vi "Obtain Broadcast Events.vi"(8 "error in (no error)":errorcluster, 10 "Create New? (F)":bool) -> (0 "error out":errorcluster, 2 "CE14_v2 Broadcast Events":T1)   [LabVIEW 2018, in "CE14_v2.lvlib"]
doc: "This VI Obtains/Creates the Broadcast events that will be used for other modules to register to receive messages from the module that owns this VI.\n\n<b>NOTE</b>: The contents of this VI are automatically generated and modified by the <b>Tools > Delacor > DQMH</b> utilities. Consider using those utilities instead of making your own modifications to this VI.\n_____\nBased on DQMH Project Template 6.0.0.91."
uses:
  CE14_v2.lvlib
  Broadcast Events--cluster.ctl
  Did Init Argument--cluster.ctl
  Status Updated Argument--cluster.ctl
  Error Reported Argument--cluster.ctl
  Stop Argument--cluster.ctl
  Get Module Execution Status Argument--cluster.ctl
  CE14 response data Argument--cluster.ctl
  Instrument Drivers/LVdriver_CE14(eMIC)/type defs/CE14.data.ctl
  Instrument Drivers/LVdriver_CE14(eMIC)/CE14_eMIC.lvlib
panel:
  # "NOTE: The contents of this VI are automatically generated and modified by the Tools > Delacor > DQMH utilities. Consider using those utilities instead of making your own modifications to this VI."
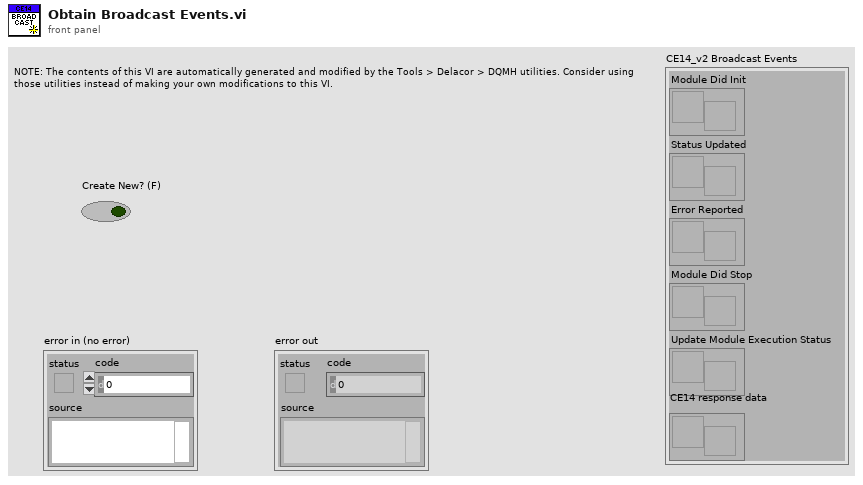
[diagram p1: front panel]
types:
  T1 = typedef "CE14_v2.lvlib/Broadcast Events--cluster.ctl" = cluster{"Module Did Init":refnum<user-event>, "Status Updated":refnum<user-event>, "Error Reported":refnum<user-event>, "Module Did Stop":refnum<user-event>, "Update Module Execution Status":refnum<user-event>, "CE14 response data":refnum<user-event>}
  T2 = typedef "CE14_v2.lvlib/CE14 response data Argument--cluster.ctl" = cluster{"Module ID":i32, "Array":T3[]}
  T3 = typedef "CE14_eMIC.lvlib/CE14.data.ctl" = cluster{"string":string, "float":dbl, "Name":string}
  T4 = typedef "CE14_v2.lvlib/Get Module Execution Status Argument--cluster.ctl" = cluster{"Module ID":i32, "Running?":bool}
  T5 = typedef "CE14_v2.lvlib/Stop Argument--cluster.ctl" = cluster{"Module ID":i32, "Origin":string, "Exit via Stop Module Req?":bool, "Wait for Module to stop?":bool}
  T6 = typedef "CE14_v2.lvlib/Error Reported Argument--cluster.ctl" = cluster{"Error":errorcluster, "Additional Information":string, "Module ID":i32, "Module Name":string}
  T7 = typedef "CE14_v2.lvlib/Status Updated Argument--cluster.ctl" = cluster{"Status":string, "Module ID":i32}
  T8 = typedef "CE14_v2.lvlib/Did Init Argument--cluster.ctl" = cluster{"Init?":bool, "Info":string, "Module ID":i32}
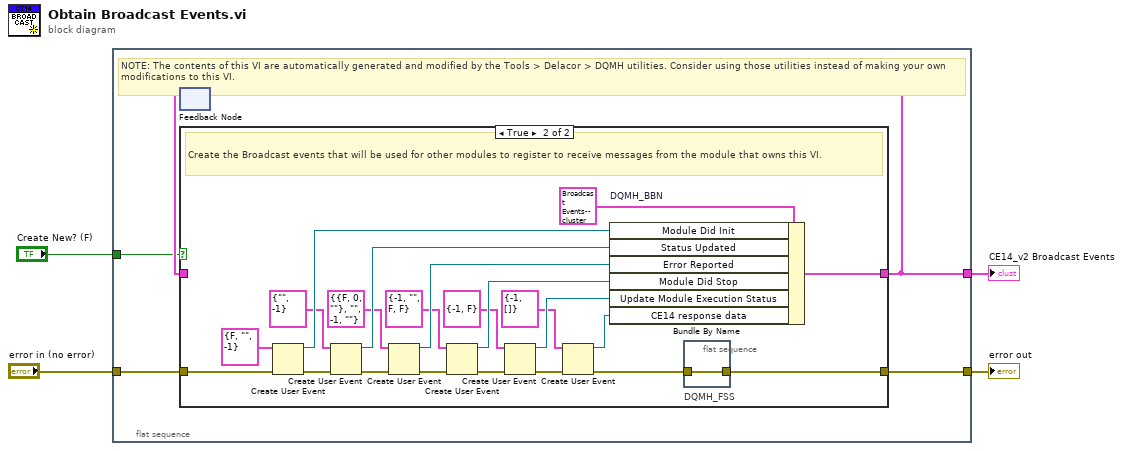
[diagram p0: block diagram]
diagram:
  n1 = flat-sequence {
    tunnel: [w9] -> w4
    tunnel: "error in (no error)" -> [w8]
    tunnel: [w6] -> w2
    tunnel: "Create New? (F)" -> [w5]
    frame #0 {
      # "NOTE: The contents of this VI are automatically generated and modified by the Tools > Delacor > DQMH utilities. Consider using those utilities instead of making your own modifications to this VI."
      n2 = feedback #1() -> (w7:T1)  [unwired: 1 in]
      n3 = case shown="True" w5 {
        tunnel: [w10 w18] -> w9
        tunnel: w8 -> [w10 w33]
        tunnel: [w11 w30] -> w6
        tunnel: w7 -> [w11 _]
        frame False {
          # "Obtain the Broadcast events that were created in a previous call to this VI."
        }
        frame True {
          # "Create the Broadcast events that will be used for other modules to register to receive messages from the module that owns this VI."
          n4 = Create User Event(user event datatype=T8 {"Init?"=FALSE, "Info"="", "Module ID"=-1} ("Did Init Argument"), error in=w33) -> (user event=w31:refnum<user-event>, error out=w28:errorcluster)
          n5 = Create User Event(user event datatype=T7 {"Status"="", "Module ID"=-1} ("Status Updated Argument"), error in=w28) -> (user event=w25:refnum<user-event>, error out=w27:errorcluster)
          n6 = Create User Event(user event datatype=T6 {"Error"={"status"=FALSE, "code"=0, "source"=""}, "Additional Information"="", "Module ID"=-1, "Module Name"=""} ("Error Reported Argument"), error in=w27) -> (user event=w22:refnum<user-event>, error out=w24:errorcluster)
          n7 = Create User Event(user event datatype=T5 {"Module ID"=-1, "Origin"="", "Exit via Stop Module Req?"=FALSE, "Wait for Module to stop?"=FALSE} ("Stop Argument"), error in=w24) -> (user event=w20:refnum<user-event>, error out=w19:errorcluster)
          n8 = Create User Event(user event datatype=T4 {"Module ID"=-1, "Running?"=FALSE} ("Get Module Execution Status Argument"), error in=w19) -> (user event=w16:refnum<user-event>, error out=w17:errorcluster)
          n9 = Create User Event(user event datatype=T2 {"Module ID"=-1, "Array"=[]} ("CE14 response data Argument"), error in=w17) -> (user event=w13:refnum<user-event>, error out=w14:errorcluster)
          n10 = Bundle By Name "DQMH_BBN"(cluster=T1 {"Module Did Init"=refnum, "Status Updated"=refnum, "Error Reported"=refnum, "Module Did Stop"=refnum, "Update Module Execution Status"=refnum, "CE14 response data"=refnum} ("output cluster"), "Module Did Init"=w31, "Status Updated"=w25, "Error Reported"=w22, "Module Did Stop"=w20, "Update Module Execution Status"=w16, "CE14 response data"=w13) -> (w30:T1)
          n11 = flat-sequence "DQMH_FSS" {
            tunnel: w14 -> [w34]
            tunnel: [w34] -> w18
            frame #0 {
            }
          }
        }
      }
      n12 = feedback-in #1(w6) -> ()
    }
  }
  "CE14_v2 Broadcast Events" <- w2
  "error out" <- w4
